vi "ElevEncActions.vi"(10 "Update?":bool, 11 "Zero?":bool) -> (3 "ElevEncPos":i32)   [LabVIEW 2018]
uses:
  <vilib>/Rock Robotics/WPI/ThirdParty/Phoenix-LabVIEW/Motor Controller/Get/CTRE_Phoenix_MotorController_GetQuadratureData.vi
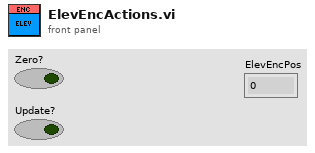
[diagram p1: front panel]
types:
  T1 = typedef "WPI_MotorControlDeviceRef.ctl" = cluster{"DeviceStatus":errorcluster, "Type":T2, "PWM":cluster{"PWM Channel":T3, "DeadBand":T4}, "CAN":cluster{"Device Number":u8, "SetOutput VI Ref":variant, "GetOutput VI Ref":variant, "Enable VI Ref":variant, "Disable VI Ref":variant, "Data":variant}, "Invert":bool, "DIO PWM":cluster{"PWM \"Enable\" Channel":T3, "DIOChannel":T5, "PWM Rate":dbl}}
  T2 = typedef "WPI_MotorControlType.ctl" = enum16{"PWM", "CAN", "DIO PWM"}
  T3 = typedef "FPGA_DIOPWMChannel.ctl" = enum8{"PWM 0", "PWM 1", "PWM 2", "PWM 3", "PWM 4", "PWM 5", "PWM 6", "PWM 7", "PWM 8", "PWM 9", "PWM MXP 0", "PWM MXP 1", "PWM MXP 2", "PWM MXP 3", "PWM MXP 4", "PWM MXP 5", "PWM MXP 6", "PWM MXP 7", "PWM MXP 8", "PWM MXP 9", "Invalid"}
  T4 = typedef "WPI_PWMDeadband.ctl" = cluster{"Name":string, "maxPositivePwm":i32, "minPositivePwm":i32, "centerPwm":i32, "maxNegativePwm":i32, "minNegativePwm":i32, "angularRange":u16}
  T5 = typedef "FPGA_DIOChannel.ctl" = enum8{"DIO 0", "DIO 1", "DIO 2", "DIO 3", "DIO 4", "DIO 5", "DIO 6", "DIO 7", "DIO 8", "DIO 9", "DIO MXP 0", "DIO MXP 1", "DIO MXP 2", "DIO MXP 3", "DIO MXP 4", "DIO MXP 5", "DIO MXP 6", "DIO MXP 7", "DIO MXP 8", "DIO MXP 9", "DIO MXP 10", "DIO MXP 11", "DIO MXP 12", "DIO MXP 13", "DIO MXP 14", "DIO MXP 15", "SPI Port CS1", "SPI Port CS2", "SPI Port CS3", "SPI Port MISO", "SPI Port MOSI", "Invalid"}
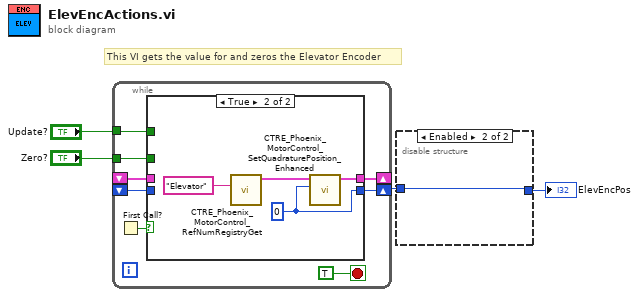
[diagram p0: block diagram]
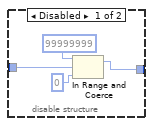
[diagram p2: hidden frame]
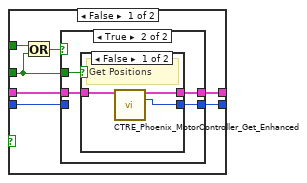
[diagram p3: hidden frame]
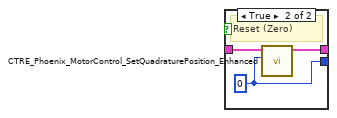
[diagram p5: hidden frame]
diagram:
  # "This VI gets the value for and zeros the Elevator Encoder"
  n1 = while {
    shift-right: [w11] -> _
    shift-left: _ -> [w10]
    tunnel: "Zero?" -> [w7]
    tunnel: "Update?" -> [w6]
    shift-right: [w12] -> w2
    shift-left: _ -> [w5]
    stop <- TRUE stop-if-true
    n2 = First Call?() -> (First Call?: T/F=w9:bool)
    n3 = case shown="True" w9 {
      tunnel: w10 -> [w19 _]
      tunnel: [w18 w32] -> w12
      tunnel: [w17 w33] -> w11
      tunnel: w7 -> [w13 _]
      tunnel: w6 -> [w14 _]
      tunnel: w5 -> [w15 _]
      frame False {
        n4 = Or(x=w14, y=w13) -> (x .or. y?=w16:bool)
        n5 = case shown="True" w16 {
          tunnel: w19 -> [w21 w25]
          tunnel: [w20 w24] -> w18
          tunnel: [w21 w23] -> w17
          tunnel: w13 -> [_ w22]
          tunnel: w15 -> [w20 _]
          frame False {
          }
          frame True {
            n6 = case shown="False" w22 {
              tunnel: w25 -> [w28 w31]
              tunnel: [w27 w29] -> w24
              tunnel: [w26 w30] -> w23
              frame False {
                # "Get Positions"
                n7 = call-poly <vilib>:"CTRE_Phoenix_MotorController_Get_Enhanced.vi"("PhoenixMotorControlDevRef"=w28) -> ("PhoenixMotorControlDevRef"=w26:T1, "Quadrature Position"=w27:i32)  [unwired: 11 in, 2 out]
              }
              frame True {
                w29 = 0 ("New Position")
                # "Reset (Zero)"
                n8 = call <vilib>:"CTRE_Phoenix_MotorControl_SetQuadraturePosition_Enhanced.vi"("New Position"=w29, "PhoenixMotorControlDevRef"=w31) -> ("PhoenixMotorControlDevRef"=w30:T1)  [unwired: 8 in, 1 out]
              }
            }
          }
        }
      }
      frame True {
        w32 = 0 ("New Sensor Position")
        n9 = call <vilib>:"CTRE_Phoenix_MotorControl_RefNumRegistryGet.vi"("refnum name"="Elevator") -> ("PhoenixMotorControlDevRef"=w34:T1)  [unwired: 9 in, 1 out]
        n10 = call <vilib>:"CTRE_Phoenix_MotorControl_SetQuadraturePosition_Enhanced.vi"("New Position"=w32, "PhoenixMotorControlDevRef"=w34) -> ("PhoenixMotorControlDevRef"=w33:T1)  [unwired: 8 in, 1 out]
      }
    }
  }
  n11 = disable-structure shown="Enabled" {
    disable-tunnel: w2 -> [w39 w40]
    disable-tunnel: [w36 w40] -> w1
    frame Disabled {
      n12 = In Range and Coerce(upper limit=99999999, x=w39, lower limit=0) -> (coerced(x)=w36:i32)  [unwired: 1 out]
    }
    frame Enabled {
    }
  }
  "ElevEncPos" <- w1
